vi "From Serial Form.vi"(6 "Serial Version":T1, 10 "Deserializer in":refnum<class "Deserializer.lvclass">, 11 "CRDS in":refnum<class "CRDS.lvclass">) -> (0 "error out":errorcluster, 2 "Deserializer out":refnum<class "Deserializer.lvclass">, 3 "CRDS out":refnum<class "CRDS.lvclass">)   [LabVIEW 2012]
uses:
  <userlib>/Serialization/Serializable/Serializable.lvclass
  Cell/CRDS Cell.lvclass
  Data/Main/CRDS Data.lvclass
  Data/Cell/CRDS Cell Data.lvclass
  <userlib>/Serialization/Serializable/Remove Boolean.vi
  <userlib>/Serialization/Serialization Common/Serial Version.ctl
  <userlib>/Serialization/Serialization Common/Serialization Common.lvlib
  <userlib>/Serialization/Deserializer/Deserializer.lvclass
  CRDS.lvclass
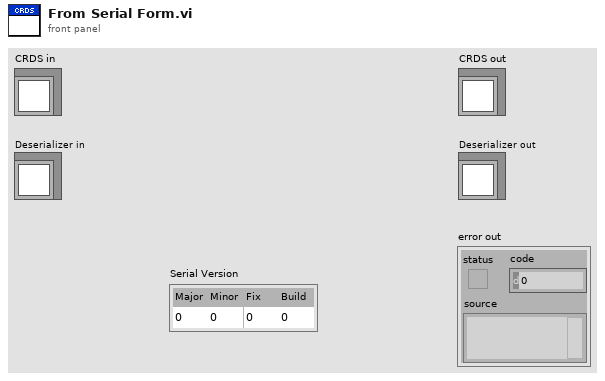
[diagram p1: front panel]
types:
  T1 = typedef "Serialization Common.lvlib/Serial Version.ctl" = cluster{"Major":u16, "Minor":u16, "Fix":u16, "Build":u16}
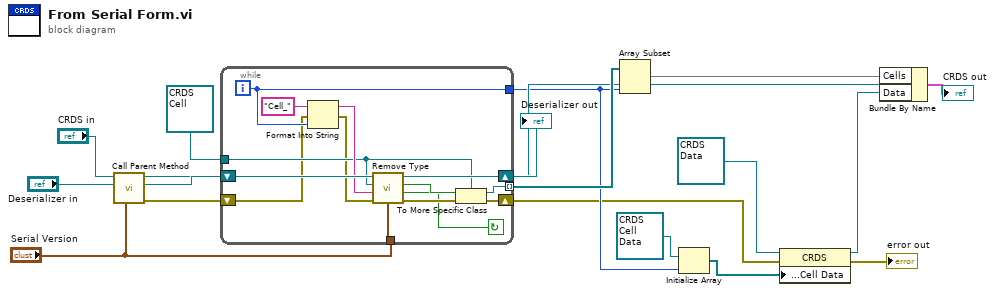
[diagram p0: block diagram]
diagram:
  n1 = call-parent "Call Parent Method"("Serial Version"="Serial Version", "Deserializer in"="Deserializer in", "Instrument in"="CRDS in") -> ("error out"=w15:errorcluster, "Deserializer out"=w16:refnum<class "Deserializer.lvclass">, "Instrument out"=w8:refnum<class "CRDS.lvclass">)  [unwired: 6 in]
  n2 = while {
    shift-right: [w25] -> w3
    shift-left: w15 -> [w20]
    tunnel: refnum<class "CRDS Cell.lvclass"> refnum ("CRDS Cell.lvclass") -> [w27]
    tunnel: [w26] -> w10 mode=indexing
    tunnel: [w22] -> w7
    tunnel: "Serial Version" -> [w21]
    shift-right: [w31] -> w13
    shift-left: w16 -> [w29]
    i -> [w22]
    stop <- w23 continue-if-true
    n3 = Format Into String(initial string="Cell_", error in=w20, w22) -> (resulting string=w30:string, error out=w19:errorcluster)  [unwired: 1 in]
    n4 = call-poly <userlib>:"Remove Type.vi"(6:w21, "error in (no error)"=w19, "Name"=w30, "Default Value"=w27, "Deserializer in"=w29) -> ("error out"=w24:errorcluster, "Found?"=w23:bool, "Boolean"=w28:bool, "Deserializer out"=w31:refnum<class "Deserializer.lvclass">)  [unwired: 3 in]
    n5 = To More Specific Class(target class=w27, reference=w28, error in=w24) -> (specific class reference=w26:refnum<class "CRDS Cell.lvclass">, error out=w25:errorcluster)
  }
  "Deserializer out" <- w13
  n6 = Array Subset(array=w10, length=w7) -> (w9:refnum<class "CRDS Cell.lvclass">[])  [unwired: 1 in]
  n7 = Initialize Array(refnum<class "CRDS Cell Data.lvclass"> refnum ("Base CRDS Lib.lvlib:CRDS Cell"), w7) -> (w4:refnum<class "CRDS Cell Data.lvclass">[])
  n8 = property class="CRDS"(reference=refnum<class "CRDS Data.lvclass"> refnum ("Data"), error in=w3, "Data Access:Cell Data"=w4) -> (reference out=w1:refnum<class "CRDS Data.lvclass">, error out=→"error out":errorcluster)
  n9 = Bundle By Name(cluster=w8, "Cells"=w9, "Data"=w1) -> (→"CRDS out":cluster{})
